vi "Create Response.vi"(8 "error in (no error)":errorcluster, 9 "body":string, 10 "headers":string, 11 "http-client":refnum<class "http-client.lvclass">) -> (0 "error out":errorcluster, 2 "response":refnum<class "response.lvclass">, 3 "http-client out":refnum<class "http-client.lvclass">)   [LabVIEW 2020, in "http.lvlib" / "http-client.lvclass"]
uses:
  http-client.lvclass
  response/response.lvclass
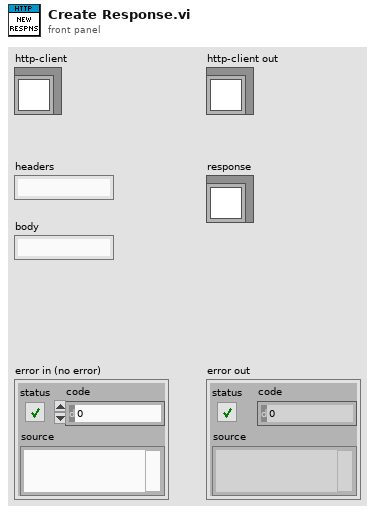
[diagram p1: front panel]
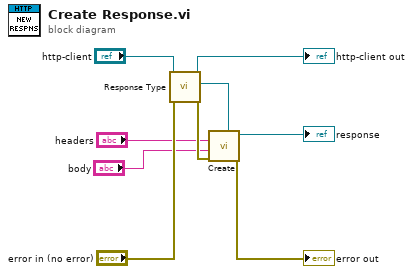
[diagram p0: block diagram]
diagram:
  n1 = call-dynamic "Response Type.vi"("error in (no error)"="error in (no error)", "http-client in"="http-client") -> ("error out"=w7:errorcluster, "response type"=w5:refnum<class "response.lvclass">, "http-client out"=→"http-client out":refnum<class "http-client.lvclass">)  [unwired: 7 in]
  n2 = call-dynamic "Create.vi"("response (type)"=w5, "error in (no error)"=w7, "body"="body", "headers"="headers") -> ("error out"=→"error out":errorcluster, "response out"=→"response":refnum<class "response.lvclass">)  [unwired: 6 in]
